vi "Convert to Coordinates.vi"(10 "Filtered Data (First Filter)":T2(array[cluster])) -> (2 "Coordinates":T1(array[cluster]))   [LabVIEW 2017]
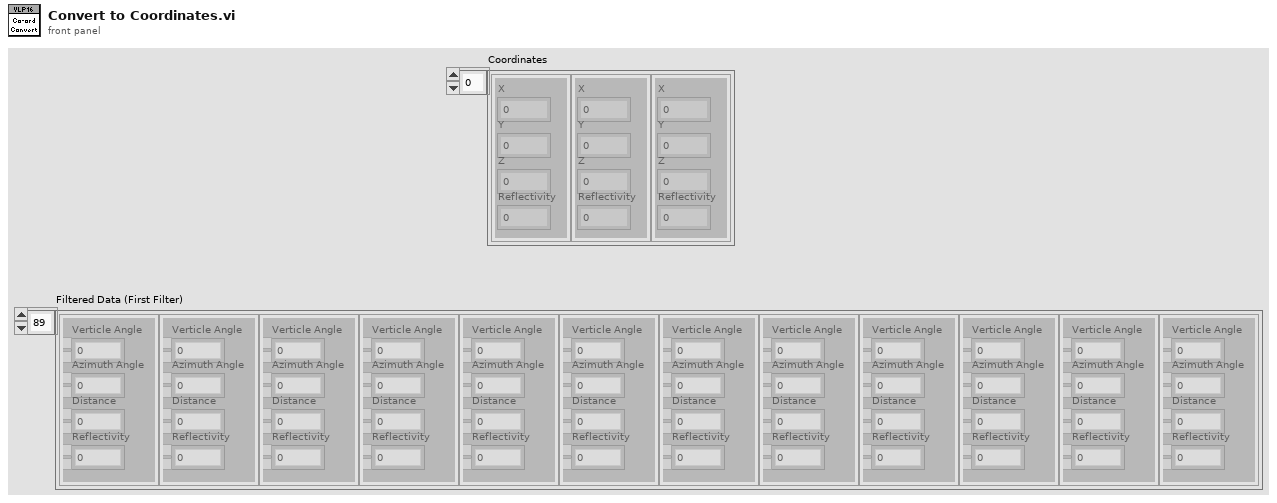
[diagram p1: front panel]
types:
  T1 = cluster{"X":dbl, "Y":dbl, "Z":dbl, "Reflectivity":dbl}[]
  T2 = cluster{"Verticle Angle":dbl, "Azimuth Angle":dbl, "Distance":dbl, "Reflectivity":dbl}[]
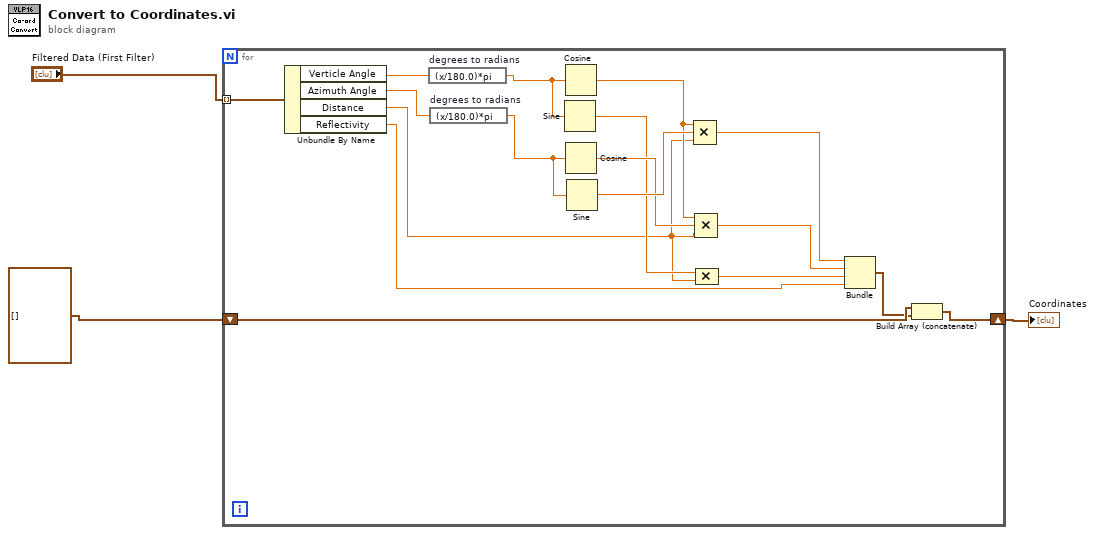
[diagram p0: block diagram]
diagram:
  n1 = for {
    shift-right: [w4] -> w1
    shift-left: cluster{dbl, dbl, dbl, dbl}[] [] -> [w6]
    tunnel: "Filtered Data (First Filter)" -> [w20] mode=indexing
    n2 = Unbundle By Name(w20) -> ("Verticle Angle"=w19:dbl, "Azimuth Angle"=w18:dbl, "Distance"=w11:dbl, "Reflectivity"=w7:dbl)
    n3 = expression code="(x/180.0)*pi" "degrees to radians"(w19) -> (w17:dbl)
    n4 = expression code="(x/180.0)*pi" "degrees to radians"(w18) -> (w16:dbl)
    n5 = Sine(x=w17) -> (sin(x)=w12:dbl)
    n6 = Cosine(x=w17) -> (cos(x)=w14:dbl)
    n7 = Cosine(x=w16) -> (cos(x)=w13:dbl)
    n8 = Sine(x=w16) -> (sin(x)=w15:dbl)
    n9 = Compound Arithmetic op=MULTIPLY(w14, w15, w11) -> (w10:dbl)
    n10 = Compound Arithmetic op=MULTIPLY(w14, w13, w11) -> (w9:dbl)
    n11 = Compound Arithmetic op=MULTIPLY(w12, w11) -> (w8:dbl)
    n12 = Bundle(w10, w9, w8, "Reflectivity"=w7) -> (w5:cluster{dbl, dbl, dbl, "Reflectivity":dbl})  [unwired: 1 in]
    n13 = Build Array (concatenate)(w6, w5) -> (w4:cluster{dbl, dbl, dbl, "Reflectivity":dbl}[])
  }
  "Coordinates" <- w1
